vi "Create.vi"(8 "error in (no error)":errorcluster) -> (0 "error out":errorcluster, 3 "CT-Energize-Cmd.lvclass":refnum<class "CT-Energize-Cmd.lvclass">)   [LabVIEW 2013, in "CT-Energize-Cmd.lvclass"]
uses:
  CT-Energize-Cmd.lvclass
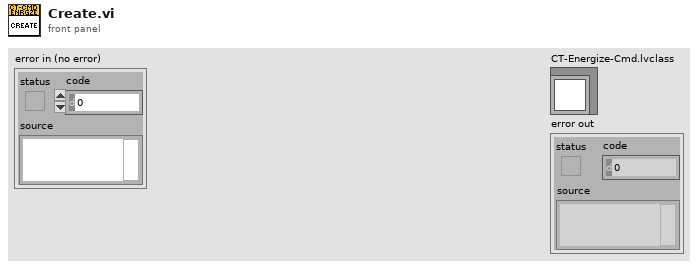
[diagram p1: front panel]
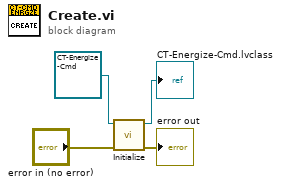
[diagram p0: block diagram]
diagram:
  n1 = call-dynamic "Initialize.vi"("error in (no error)"="error in (no error)", "CT-Energize-Cmd in"=refnum<class "CT-Energize-Cmd.lvclass"> refnum ("CT-Energize-Cmd.lvclass")) -> ("error out"=→"error out":errorcluster, "CT-Energize-Cmd out"=→"CT-Energize-Cmd.lvclass":refnum<class "CT-Energize-Cmd.lvclass">)  [unwired: 8 in]
